vi "Practica 2 Operaciones Basicas con Arrays Multiplicacion.vi"() -> ()   [LabVIEW 2016]
panel:
  out "Result":dbl[][](array[numeric])
  in  "Matriz Inversa":dbl[][](array[numeric])
  in  "Matriz de Coeficientes":dbl[][](array[numeric])
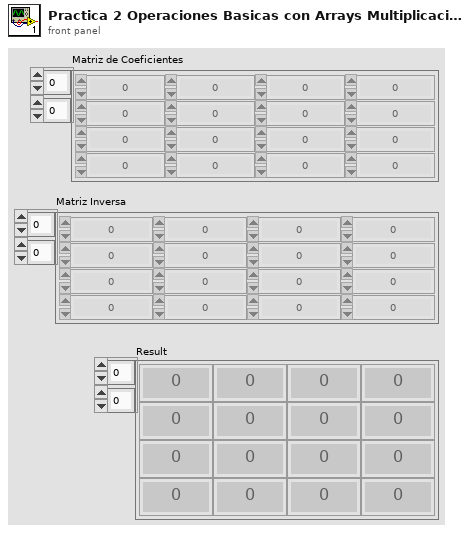
[diagram p1: front panel]
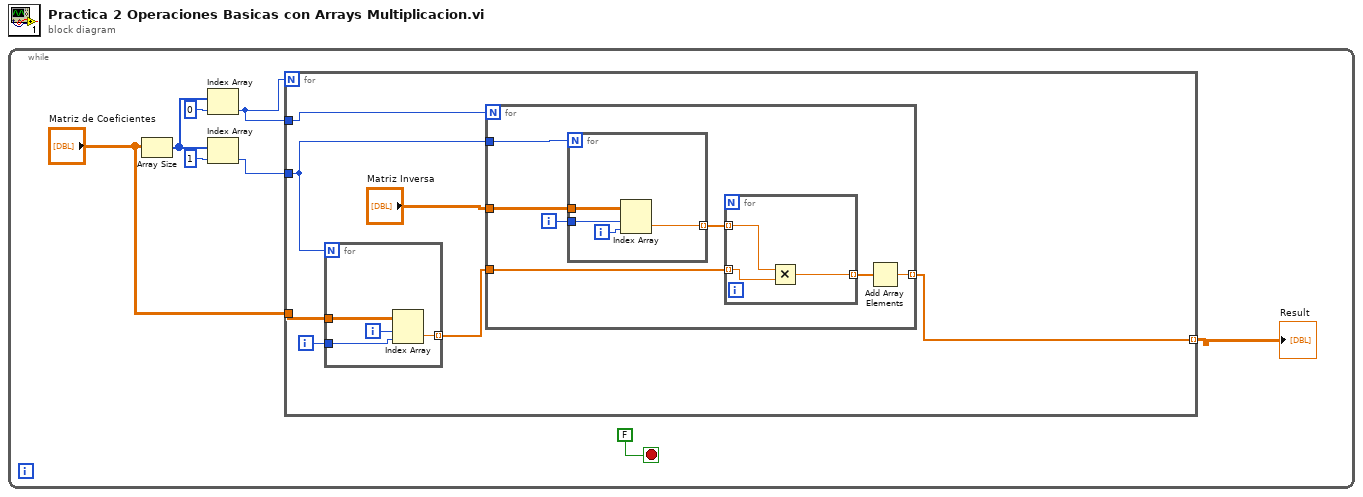
[diagram p0: block diagram]
diagram:
  n1 = while {
    stop <- FALSE stop-if-true
    n2 = Array Size(array="Matriz de Coeficientes") -> (size(s)=w7:i32[])
    n3 = Index Array(array=w7, index=0) -> (element=w3:i32)
    n4 = Index Array(array=w7, index=1) -> (element=w5:i32)
    n5 = for {
      N: w3 -> [_]
      tunnel: "Matriz de Coeficientes" -> [w15]
      tunnel: w5 -> [w13]
      tunnel: [w11] -> w1 mode=indexing
      tunnel: w3 -> [w10]
      i -> [w14]
      n6 = for {
        N: w13 -> [_]
        tunnel: w15 -> [w33]
        tunnel: [w32] -> w12 mode=indexing
        tunnel: w14 -> [w30]
        i -> [w31]
        n7 = Index Array(array=w33, index (row)=w31, index (col)=w30) -> (element=w32:dbl)
      }
      n8 = for {
        N: w10 -> [_]
        tunnel: "Matriz Inversa" -> [w21]
        tunnel: w13 -> [w20]
        tunnel: w12 -> [w19]
        tunnel: [w17] -> w11 mode=indexing
        i -> [w16]
        n9 = for {
          N: w20 -> [_]
          tunnel: w21 -> [w26]
          tunnel: w16 -> [w25]
          tunnel: [w23] -> w18 mode=indexing
          i -> [w24]
          n10 = Index Array(array=w26, index (row)=w25, index (col)=w24) -> (element=w23:dbl)
        }
        n11 = for {
          tunnel: w19 -> [w27] mode=indexing
          tunnel: w18 -> [w28] mode=indexing
          tunnel: [w29] -> w22 mode=indexing
          n12 = Multiply(x=w28, y=w27) -> (x*y=w29:dbl)
        }
        n13 = Add Array Elements(numeric array=w22) -> (sum=w17:dbl)
      }
    }
    "Result" <- w1
  }
